vi "MB1010AnalogPID.vi"(5 "output range (100, -100)":cluster{"output high":dbl, "output low":dbl}={"output high"=100.0, "output low"=-100.0} {"output low" format="%.2f"; "output high" format="%.2f"}, 7 "PID gains":T4={"proportional gain (Kc)"=1.0, "integral time (Ti, min)"=0.01, "derivative time (Td, min)"=0.0} {"derivative time (Td, min)" format="%.3f"; "integral time (Ti, min)" format="%.3f"; "proportional gain (Kc)" format="%.3f"}, 8 "error in (no error)":errorcluster, 9 "FullSpeed":bool, 10 "setpoint":dbl format="%.2f", 11 "AIDeviceRef":T1) -> (0 "error out":errorcluster, 1 "CrossedSetpoint":bool, 2 "output":dbl, 3 "AIDeviceRef":T1)   [LabVIEW 2013]
uses:
  <vilib>/Rock Robotics/WPI/AnalogChannel/WPI_AnalogChannelDevRef.ctl
  <vilib>/Rock Robotics/SystemInterfaces/Typedef/FPGA_TypedefAnalogModule.ctl
  <vilib>/Rock Robotics/SystemInterfaces/AI/FPGA_AIChannel.ctl
  <vilib>/addons/control/pid/pid.llb/PID Control Input Filter (DBL).vi
  <vilib>/addons/control/pid/pid.llb/PID (DBL).vi
  <vilib>/addons/control/pid/NI_PID_pid.lvlib
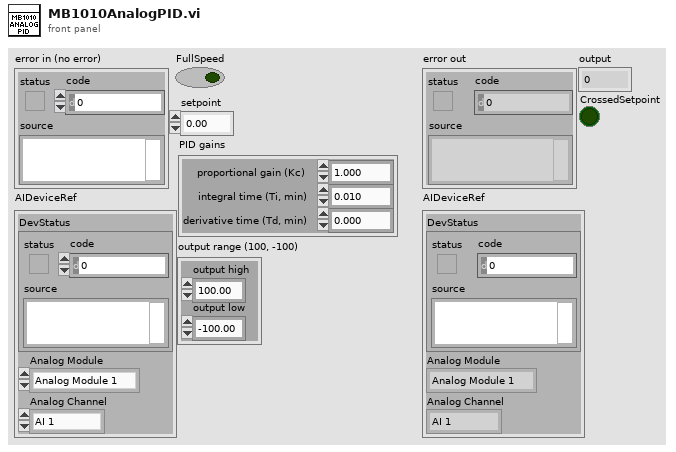
[diagram p1: front panel]
types:
  T1 = typedef "WPI_AnalogChannelDevRef.ctl" = cluster{"DevStatus":errorcluster, "Analog Module":T2, "Analog Channel":T3}
  T2 = typedef "FPGA_TypedefAnalogModule.ctl" = enum16{"Analog Module 1", "Analog Module 2"}
  T3 = typedef "FPGA_AIChannel.ctl" = enum8{"AI 1", "AI 2", "AI 3", "AI 4", "AI 5", "AI 6", "AI 7", "AI 8", "Invalid"}
  T4 = cluster{"proportional gain (Kc)":dbl, "integral time (Ti, min)":dbl, "derivative time (Td, min)":dbl}
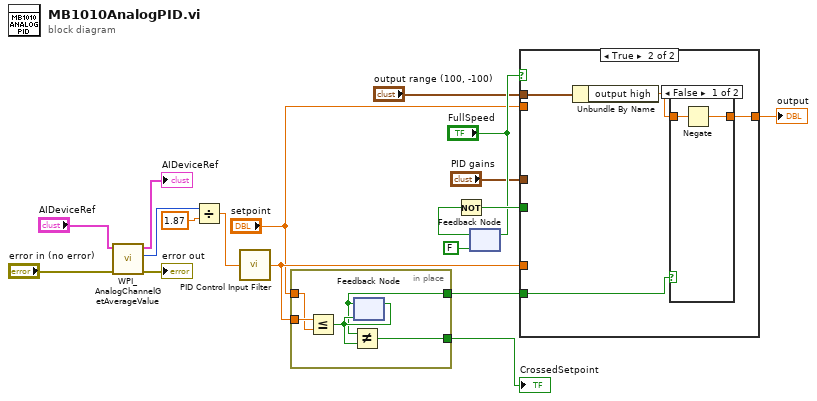
[diagram p0: block diagram]
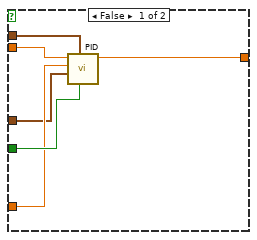
[diagram p2: hidden frame]
diagram:
  n1 = call <vilib>:"WPI_AnalogChannelGetAverageValue.vi"("error in (no error)"="error in (no error)", "AIDeviceRef"="AIDeviceRef") -> ("error out"=→"error out":errorcluster, "Value"=w18:i32, "AIDeviceRef"=→"AIDeviceRef":T1)  [unwired: 7 in]
  n2 = Divide(x=w18, y=1.87 ("scaling factor")) -> (x/y=w17:dbl)
  n3 = call-poly <vilib>:"PID Control Input Filter.vi"("input"=w17) -> ("output"=w12:dbl)  [unwired: 4 in]
  n4 = in-place {
    in-place-border: w12 -> [w23]
    in-place-border: [w22] -> w1
    in-place-border: [w20] -> w11
    in-place-border: "setpoint" -> [w19]
    n5 = Less Or Equal?(x=w23, y=w19) -> (x <= y?=w21:bool)
    n6 = feedback #1(w21) -> (w20:bool)
    n7 = Not Equal?(x=w20, y=w21) -> (x != y?=w22:bool)
    n8 = feedback-in #1(w21) -> ()
  }
  "CrossedSetpoint" <- w1
  n9 = feedback #2(FALSE) -> (w13:bool)
  n10 = Not(x=w13) -> (.not. x?=w14:bool)
  n11 = feedback-in #2("FullSpeed") -> ()
  n12 = case shown="True" "FullSpeed" {
    tunnel: w14 -> [w29 _]
    tunnel: [w28 w33] -> w3
    tunnel: w12 -> [w27 _]
    tunnel: w11 -> [_ w32]
    tunnel: "setpoint" -> [w26 _]
    tunnel: "output range (100, -100)" -> [w25 w31]
    tunnel: "PID gains" -> [w24 _]
    frame False {
      n13 = call-poly <vilib>:"PID.vi"("reinitialize? (F)"=w29, "output range"=w25, "PID gains"=w24, "process variable"=w27, "setpoint"=w26) -> ("output"=w28:dbl)  [unwired: 5 in, 1 out]
    }
    frame True {
      n14 = Unbundle By Name(w31) -> ("output high"=w30:dbl)
      n15 = case shown="False" w32 {
        tunnel: [w35 w36] -> w33
        tunnel: w30 -> [w34 w36]
        frame False {
          n16 = Negate(x=w34) -> (-x=w35:dbl)
        }
        frame True {
        }
      }
    }
  }
  "output" <- w3
